vi "Init Error MsgBox.vi"(4 "Show Details? (F)":bool, 6 "Allow to close? (T)":bool=TRUE, 7 "Msg_Error in":refnum<class "Msg_Error.lvclass">, 8 "error in":errorcluster, 9 "Timeout (-1)":i32=-1, 10 "Call Chain":string[](array[string]), 11 "Error":errorcluster) -> (0 "error out":errorcluster, 3 "Msg_Error out":refnum<class "Msg_Error.lvclass">)   [LabVIEW 2012, in "Msg_Error.lvlib" / "Msg_Error.lvclass"]
doc: "Instantiates an object of class \"Error Message Box\"."
uses:
  Msg_Error.lvclass
  <vilib>/Utility/error.llb/DialogType.ctl
  Msg_Error.lvclass/Msg_Error.ctl
  MessageBox/MessageBox.lvclass
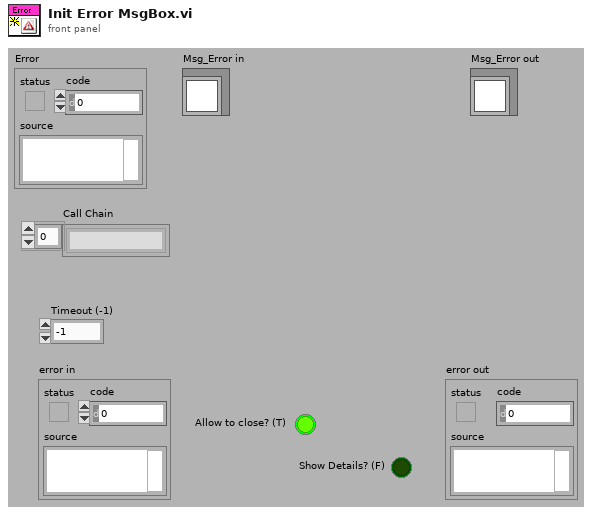
[diagram p1: front panel]
types:
  T1 = typedef "DialogType.ctl" = u16
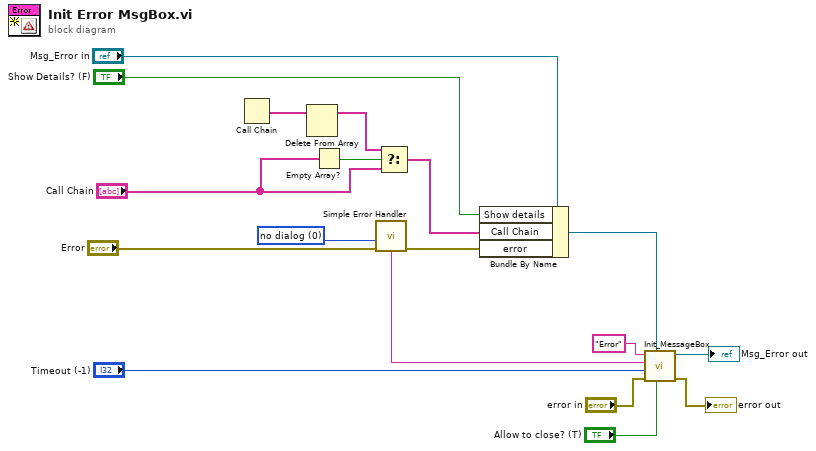
[diagram p0: block diagram]
diagram:
  w9 = T1 0 items=["no dialog", "OK message", "continue or stop message", "OK message + warnings", "continue/stop + warnings"] ("type of dialog (OK msg:1)")
  n1 = Call Chain() -> (call chain=w15:string[])
  n2 = Delete From Array(array=w15) -> (array with subset deleted=w14:string[])  [unwired: 2 in, 1 out]
  n3 = Empty Array?(array="Call Chain") -> (empty?=w17:bool)
  n4 = call <vilib>:"Simple Error Handler.vi"("type of dialog (OK msg:1)"=w9, "error in (no error)"="Error") -> ("error out"=w3:errorcluster, "message"=w4:string)  [unwired: 1 in, 5 out]
  n5 = Select(t=w14, s=w17, f="Call Chain") -> (s? t:f=w5:string[])
  n6 = Bundle By Name(cluster="Msg_Error in", "Show details"="Show Details? (F)", "Call Chain"=w5, "error"=w3) -> (w13:refnum<class "Msg_Error.lvclass">)
  n7 = call "Init_MessageBox.vi"("Allow to close? (T)"="Allow to close? (T)", "MessageBox in"=w13, "error in (no error)"="error in", "Timeout (-1)"="Timeout (-1)", "Message"=w4, "MsgBox Title"="Error") -> ("error out"=→"error out":errorcluster, "MessageBox out"=→"Msg_Error out":refnum<class "Msg_Error.lvclass">)  [unwired: 1 in, 3 out]
